vi "get_total_number_of_pixels_per_cycle.vi"(8 "error in (no error)":errorcluster, 11 "GenericTrajectory in":refnum<class "GenericTrajectory.lvclass">) -> (0 "error out":errorcluster, 2 "total number of pixels per cycle":i32, 3 "GenericTrajectory out":refnum<class "GenericTrajectory.lvclass">)   [LabVIEW 2010, in "GenericTrajectory.lvclass"]
doc: "returns the total number of pixels of one complete scan cycle/repetition"
uses:
  GenericTrajectory.lvclass
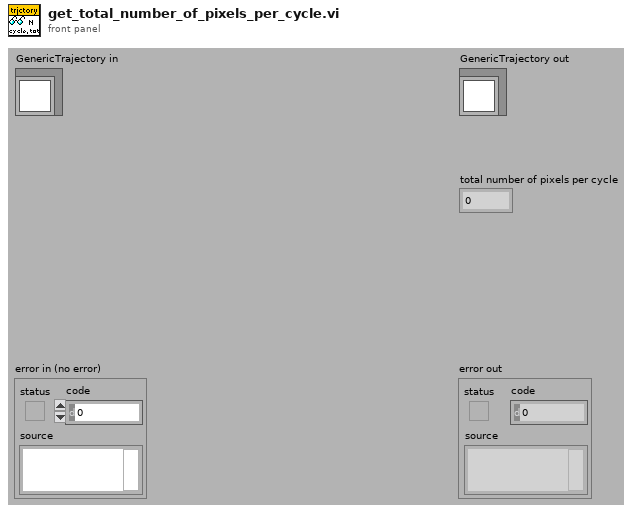
[diagram p1: front panel]
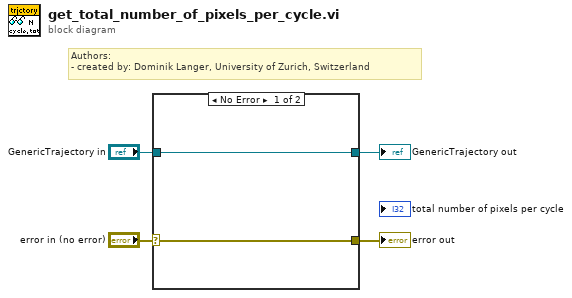
[diagram p0: block diagram]
diagram:
  # "Authors: \n- created by: Dominik Langer, University of Zurich, Switzerland"
  n1 = case shown="No Error" "error in (no error)" {
    selector: "error in (no error)" -> [w5 w8]
    tunnel: [w5 w8] -> w3
    tunnel: [w6 w7] -> w1
    tunnel: "GenericTrajectory in" -> [w6 w7]
    frame No Error {
    }
    frame Error {
    }
  }
  "error out" <- w3
  "GenericTrajectory out" <- w1
